vi "Query Measurement.vi"(8 "error in (no error)":errorcluster, 10 "States":dbl[](array[numeric]), 11 "Agilent 428x in":refnum<class "Agilent 428x.lvclass">) -> (0 "error out":errorcluster, 1 "Secondary results":dbl[](array[numeric]), 2 "Capacitances (fF)":dbl[](array[numeric]), 3 "Agilent 428x out":refnum<class "Agilent 428x.lvclass">)   [LabVIEW 2020, in "Agilent 428x.lvclass"]
uses:
  Agilent 428x.lvclass
  C:/Sandbox/RF Bench/Source Code/WiSpry Test Framework/Instruments/Instrument.lvclass
  Instrument.lvclass/Instrument.ctl
  <instrlib>/Agilent 428X Series/Agilent 428X Series.lvlib
  Instrument.lvclass
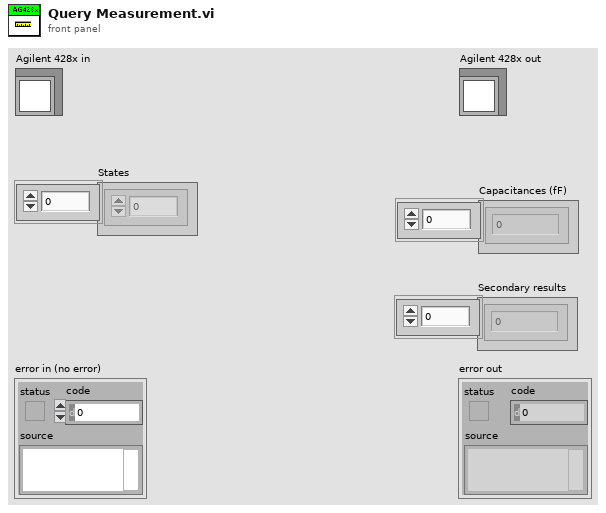
[diagram p1: front panel]
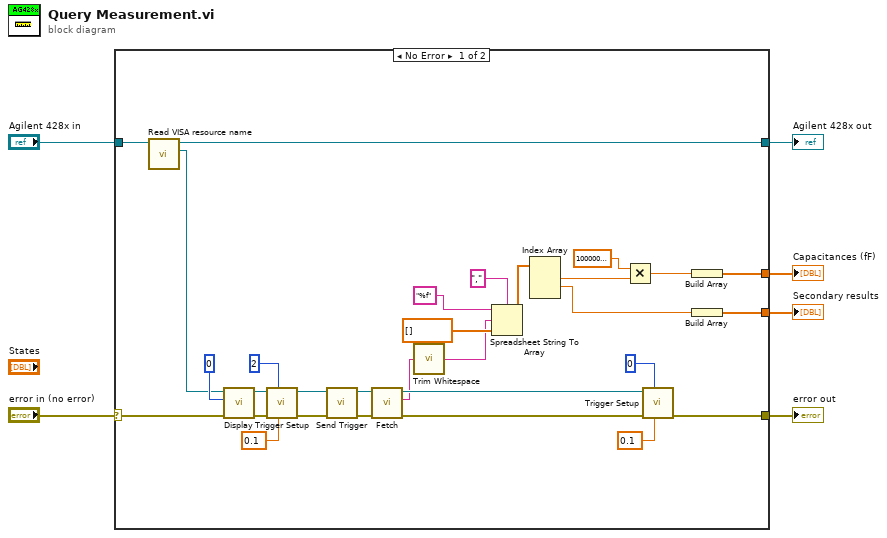
[diagram p0: block diagram]
diagram:
  n1 = case shown="No Error" "error in (no error)" {
    selector: "error in (no error)" -> [w24 w38]
    tunnel: [w23 w38] -> w5
    tunnel: [w19 w37] -> w4
    tunnel: "Agilent 428x in" -> [w20 w37]
    tunnel: [w21 _] -> w2
    tunnel: [w7 _] -> w1
    frame No Error {
      n2 = call "Read VISA resource name.vi"("Instrument in"=w20) -> ("VISA resource name"=w18:refnum<visa-resource-name>, "Instrument out"=w19:refnum<class "Agilent 428x.lvclass">)  [unwired: 9 in]
      n3 = call <instrlib>:"Display.vi"("error in (no error)"=w24, "Display Page (0: Measurement)"=u32 0 ("Display Page (Measurment:0)"), "VISA resource name"=w18) -> ("error out"=w32:errorcluster, "VISA resource name out"=w33:refnum<visa-resource-name>)  [unwired: 7 in]
      n4 = call <instrlib>:"Trigger Setup.vi"("Delay Value (s) (0.0)"=0.1, "Trigger Source (0: Internal)"=u32 2 ("Trigger Source (Internal:0)"), "error in (no error)"=w32, "VISA resource name"=w33) -> ("error out"=w26:errorcluster, "VISA resource name out"=w25:refnum<visa-resource-name>)  [unwired: 6 in]
      n5 = call <instrlib>:"Send Trigger.vi"("error in (no error)"=w26, "VISA resource name"=w25) -> ("error out"=w28:errorcluster, "VISA resource name out"=w27:refnum<visa-resource-name>)  [unwired: 8 in]
      n6 = call <instrlib>:"Fetch.vi"("error in (no error)"=w28, "VISA resource name"=w27) -> ("error out"=w17:errorcluster, "Returned Data"=w10:string, "VISA resource name out"=w16:refnum<visa-resource-name>)  [unwired: 7 in]
      n7 = call <vilib>:"Trim Whitespace.vi"("string"=w10) -> ("trimmed string"=w14:string)  [unwired: 1 in]
      n8 = Spreadsheet String To Array(delimiter (Tab)=",", format string="%f", spreadsheet string=w14, array type (2D Dbl)=dbl[] []) -> (array=w13:dbl[])
      n9 = Index Array(array=w13) -> (element #1=w9:dbl, element #2=w8:dbl)  [unwired: 3 in, 1 out]
      n10 = Multiply(x=1000000000000000.0, y=w9) -> (x*y=w22:dbl)
      n11 = call <instrlib>:"Trigger Setup.vi"("Delay Value (s) (0.0)"=0.1, "Trigger Source (0: Internal)"=u32 0 ("Trigger Source (Internal:0)"), "error in (no error)"=w17, "VISA resource name"=w16) -> ("error out"=w23:errorcluster)  [unwired: 6 in, 1 out]
      n12 = Build Array(w22) -> (w21:dbl[])
      n13 = Build Array(w8) -> (w7:dbl[])
    }
    frame Error {
    }
  }
  "error out" <- w5
  "Agilent 428x out" <- w4
  "Capacitances (fF)" <- w2
  "Secondary results" <- w1
